vi "PCO_Grab_Save.vi"(7 "# of frames":u16, 8 "entrée d'erreur (pas d'erreur)":errorcluster, 9 "Message Data":variant, 11 "Camera en entrée":refnum<class "Camera.lvclass">) -> (0 "sortie d'erreur":errorcluster, 1 "meta_data_list":T1(array[cluster]), 2 "Raw data (U16)":u16[][][](array[numeric]), 3 "Camera en sortie":refnum<class "Camera.lvclass">)   [LabVIEW 2026]
uses:
  pco.labview/camera/Camera.lvclass
  Controls/PCO_Config.ctl
panel:
  out "recorded_image_count":u32
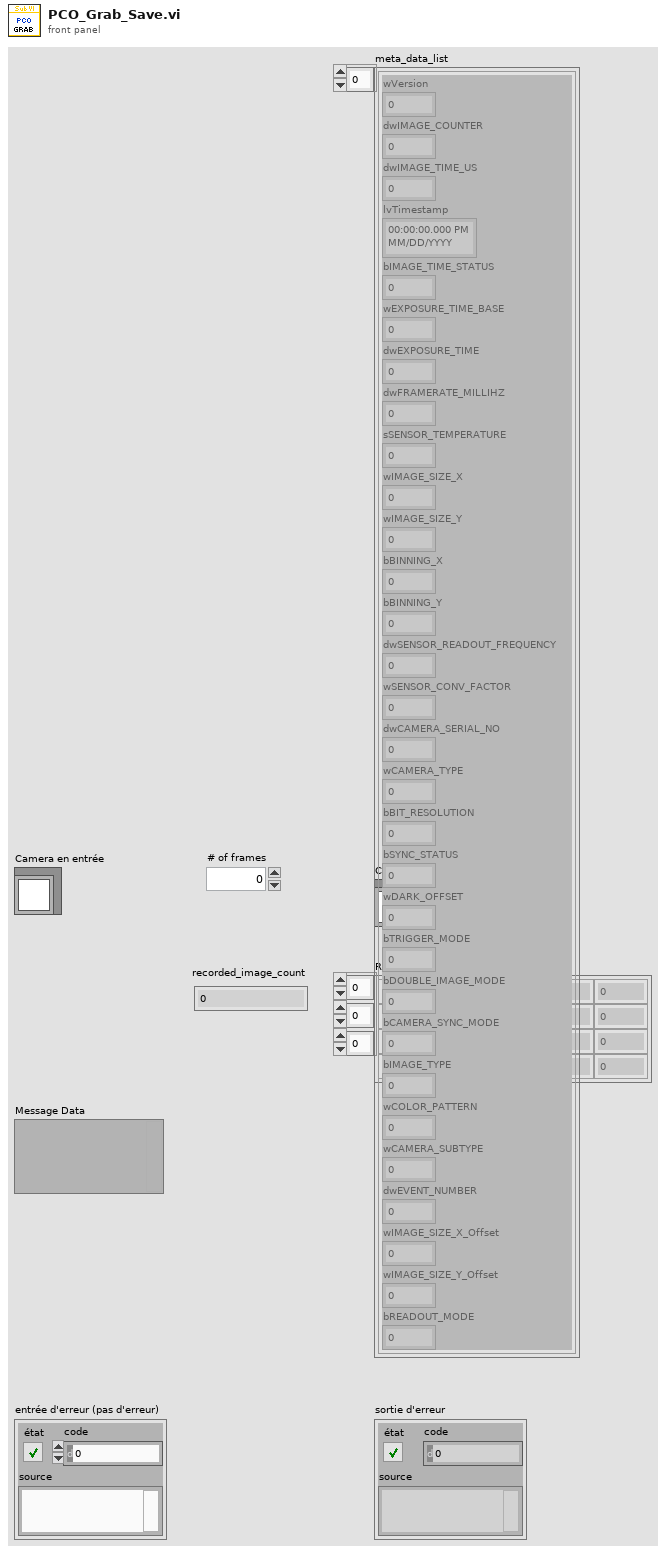
[diagram p1: front panel]
types:
  T1 = cluster{"wVersion":u16, "dwIMAGE_COUNTER":u32, "dwIMAGE_TIME_US":u32, "lvTimestamp":timestamp, "bIMAGE_TIME_STATUS":u8, "wEXPOSURE_TIME_BASE":u16, "dwEXPOSURE_TIME":u32, "dwFRAMERATE_MILLIHZ":u32, "sSENSOR_TEMPERATURE":i16, "wIMAGE_SIZE_X":u16, "wIMAGE_SIZE_Y":u16, "bBINNING_X":u8, "bBINNING_Y":u8, "dwSENSOR_READOUT_FREQUENCY":u32, "wSENSOR_CONV_FACTOR":u16, "dwCAMERA_SERIAL_NO":u32, "wCAMERA_TYPE":u16, "bBIT_RESOLUTION":u8, "bSYNC_STATUS":u8, "wDARK_OFFSET":u16, "bTRIGGER_MODE":u8, "bDOUBLE_IMAGE_MODE":u8, "bCAMERA_SYNC_MODE":u8, "bIMAGE_TYPE":u8, "wCOLOR_PATTERN":u16, "wCAMERA_SUBTYPE":u16, "dwEVENT_NUMBER":u32, "wIMAGE_SIZE_X_Offset":u16, "wIMAGE_SIZE_Y_Offset":u16, "bREADOUT_MODE":u8}[]
  T2 = enum16{"sequence", "sequence non blocking", "ring buffer", "fifo", "tif", "multitif", "pcoraw", "b16", "dicom", "multidicom", "camram_ring", "camram_segment"}
  T3 = enum16{"Undefined", "Mono8", "Mono16", "BGRA8", "RGBA8", "BGRA16", "RGBA16", "CompressedMono8"}
  T4 = typedef "PCO_Config.ctl" = cluster{"Exposure time (s)":dbl, "TriggerMode":u16, "ROI X0":u16, "ROI Y0":u16, "ROI X1":u16, "ROI Y1":u16, "Binning":u8}
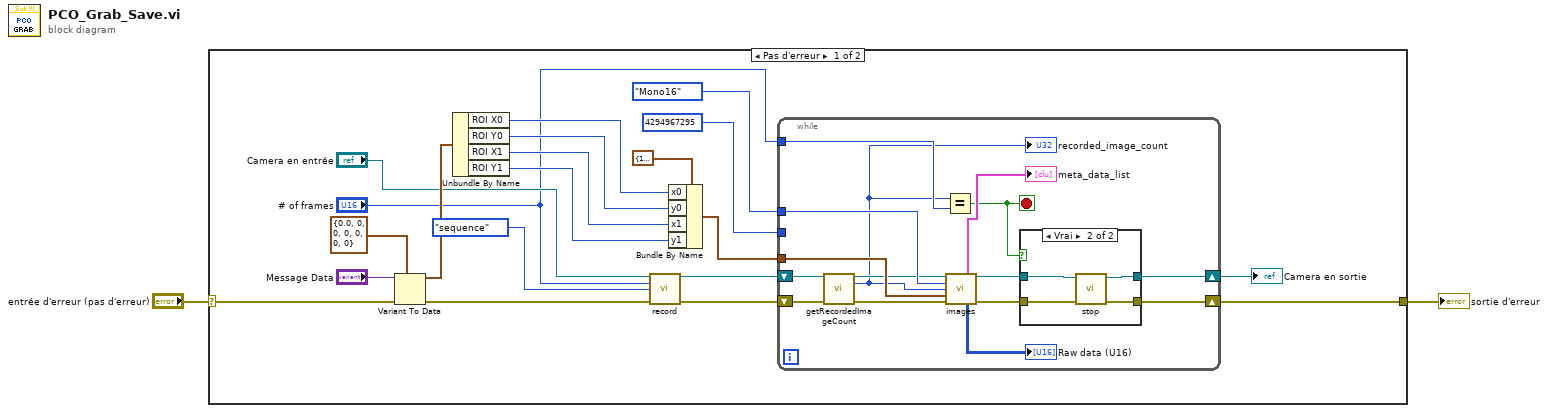
[diagram p0: block diagram]
diagram:
  n1 = case shown="Pas d'erreur" "entrée d'erreur (pas d'erreur)" {
    selector: "entrée d'erreur (pas d'erreur)" -> [w7 w44]
    tunnel: [w6 w44] -> w2
    frame No Error {
      n2 = Variant To Data(error in=w7, type=T4 {"Exposure time (s)"=0.0, "TriggerMode"=0, "ROI X0"=0, "ROI Y0"=0, "ROI X1"=0, "ROI Y1"=0, "Binning"=0} ("PCO_Config"), Variant="Message Data") -> (data=w16:T4, error out=w13:errorcluster)
      n3 = Unbundle By Name(w16) -> ("ROI X0"=w20:u16, "ROI Y0"=w19:u16, "ROI X1"=w18:u16, "ROI Y1"=w17:u16)
      n4 = call-dynamic "record.vi"("Camera in"="Camera en entrée", "num_images"="# of frames", "record_mode"=T2."sequence", "error in (no error)"=w13) -> ("Camera out"=w8:refnum<class "Camera.lvclass">, "error out"=w9:errorcluster)  [unwired: 10 in]
      n5 = Bundle By Name(cluster=cluster{"x0":u64, "y0":u64, "x1":u64, "y1":u64} {"x0"=18446744073709551615, "y0"=18446744073709551615, "x1"=18446744073709551615, "y1"=18446744073709551615} ("roi"), "x0"=w20, "y0"=w19, "x1"=w18, "y1"=w17) -> (w21:cluster{"x0":u64, "y0":u64, "x1":u64, "y1":u64})
      n6 = while {
        tunnel: T3."Mono16" ("data_format") -> [w37]
        tunnel: w21 -> [w36]
        tunnel: u32 4294967295 ("dwImgIdx") -> [_]
        shift-right: [w28] -> w6
        shift-left: w9 -> [w33]
        shift-right: [w25] -> w10
        shift-left: w8 -> [w32]
        tunnel: "# of frames" -> [w27]
        stop <- w24 stop-if-true
        n7 = call-dynamic "getRecordedImageCount.vi"("Camera in"=w32, "error in (no error)"=w33) -> ("Camera out"=w34:refnum<class "Camera.lvclass">, "recorded_image_count"=w23:u32, "error out"=w35:errorcluster)  [unwired: 11 in]
        "recorded_image_count" <- w23
        n8 = Equal?(x=w23, y=w27) -> (x = y?=w24:bool)
        n9 = call-dynamic "images.vi"("Camera in"=w34, "data_format"=w37, "image_count"=w23, "crop"=w36, "error in (no error)"=w35) -> ("meta_data_list"=→"meta_data_list":T1, "Camera out"=w26:refnum<class "Camera.lvclass">, "raw_image_list (U16)"=→"Raw data (U16)":u16[][][], "error out"=w29:errorcluster)  [unwired: 2 in, 5 out]
        n10 = case shown="Vrai" w24 {
          tunnel: w29 -> [w39 w43]
          tunnel: [w39 w42] -> w28
          tunnel: w26 -> [w38 w41]
          tunnel: [w38 w40] -> w25
          frame False {
          }
          frame True {
            n11 = call-dynamic "stop.vi"("error in (no error)"=w43, "Camera in"=w41) -> ("error out"=w42:errorcluster, "Camera out"=w40:refnum<class "Camera.lvclass">)  [unwired: 8 in]
          }
        }
      }
      "Camera en sortie" <- w10
    }
    frame Error {
    }
  }
  "sortie d'erreur" <- w2
